vi "Find Transition.vi"(0 "Tosca in":refnum<class "Parameters.lvclass">, 5 "Source":string, 7 "Target":string, 9 "Event":string, 11 "error in (no error)":errorcluster, 12 "Type":string) -> (4 "Tosca out":refnum<class "Parameters.lvclass">, 6 "stateIndex":i32, 8 "transIndex":i32, 10 "termination":bool, 15 "error out":errorcluster)   [LabVIEW 2015, in "Parameters.lvclass"]
uses:
  Parameters.lvclass
  Parameters.lvclass/Parameters.ctl
  State/State.lvclass/State.ctl
  State/Read Name.vi
  State/State.lvclass
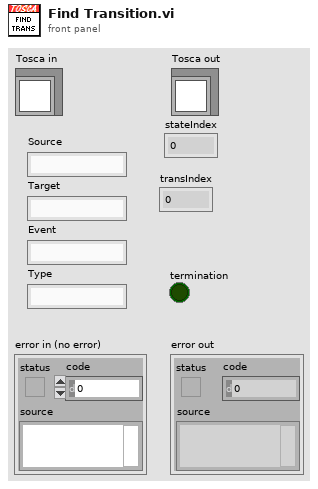
[diagram p1: front panel]
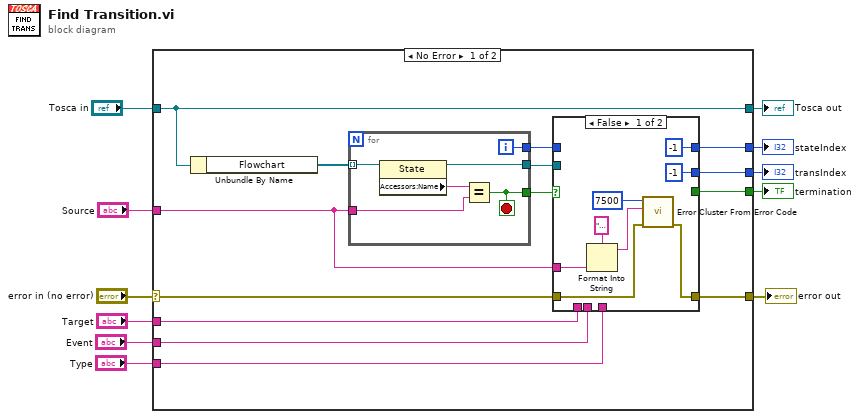
[diagram p0: block diagram]
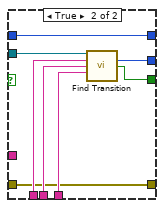
[diagram p2: hidden frame]
diagram:
  n1 = case shown="No Error" "error in (no error)" {
    selector: "error in (no error)" -> [w14 w49]
    tunnel: [w13 w49] -> w10
    tunnel: [w24 w48] -> w8
    tunnel: "Tosca in" -> [w24 w48]
    tunnel: "Source" -> [w12 _]
    tunnel: "Target" -> [w19 _]
    tunnel: "Event" -> [w18 _]
    tunnel: "Type" -> [w17 _]
    tunnel: [w22 _] -> w3
    tunnel: [w21 _] -> w2
    tunnel: [w15 _] -> w1
    frame No Error {
      n2 = Unbundle By Name(w24) -> ("Flowchart"=w25:refnum<class "State.lvclass">[])
      n3 = for {
        tunnel: w25 -> [w47] mode=indexing
        tunnel: w12 -> [w45]
        tunnel: [w44] -> w23
        tunnel: [w43] -> w16
        tunnel: [w42] -> w20
        i -> [w43]
        stop <- w42 stop-if-true
        n4 = property class="State"(reference=w47) -> (reference out=w44:refnum<class "State.lvclass">, "Accessors:Name"=w46:string)  [unwired: 1 in, 1 out]
        n5 = Equal?(x=w46, y=w45) -> (x = y?=w42:bool)
      }
      n6 = case shown="False" w20 {
        tunnel: w23 -> [_ w41]
        tunnel: [-1 ("transIndex") w40] -> w22
        tunnel: [_ w39] -> w21
        tunnel: w19 -> [_ w38]
        tunnel: w18 -> [_ w37]
        tunnel: w17 -> [_ w36]
        tunnel: w16 -> [_ w35]
        tunnel: [-1 w35] -> w15
        tunnel: w14 -> [w31 w34]
        tunnel: [w30 w34] -> w13
        tunnel: w12 -> [w26 _]
        frame False {
          n7 = Format Into String(format string="Tosca.Find Transition: source state '%s' not found" ("error message (\"\")"), w26) -> (resulting string=w27:string)  [unwired: 2 in, 1 out]
          n8 = call <vilib>:"Error Cluster From Error Code.vi"("error in (no error)"=w31, "error message (\"\")"=w27, "error code (0)"=7500) -> ("error out"=w30:errorcluster)  [unwired: 6 in]
        }
        frame True {
          n9 = call "Find Transition.vi"("State in"=w41, "Target"=w38, "Event"=w37, "Type"=w36) -> ("transIndex"=w40:i32, "termination"=w39:bool)  [unwired: 8 in, 2 out]
        }
      }
    }
    frame Error {
    }
  }
  "error out" <- w10
  "Tosca out" <- w8
  "stateIndex" <- w1
  "transIndex" <- w3
  "termination" <- w2
